vi "Pop-up Config.vi"(0 "Motor Pop-up Config":T1, 1 "Offset":T5, 2 "Motor Indicator":refnum<vi>, 3 "Motor Pop-up":refnum<vi>, 4 "VFD Pop-up":refnum<vi>, 5 "Motor_Title":refnum<vi>, 6 "Main Tab":refnum<vi>, 7 "VFD_Title":refnum<vi>, 9 "Motor Descriptions":string[](array[string]), 11 "Motor_Sel (Round)":refnum<vi>, 13 "Motor_Sel (Square)":refnum<vi>) -> ()   [LabVIEW 2020]
uses:
  <vilib>/Utility/miscctls.llb/LVPositionTypeDef.ctl
  Type Defs/Motor Pop-up Config Type Def.ctl
  Type Defs/Motors Type Def.ctl
  Type Defs/Motor Type Type Def.ctl
  Type Defs/Pop-up Corner Type Def.ctl
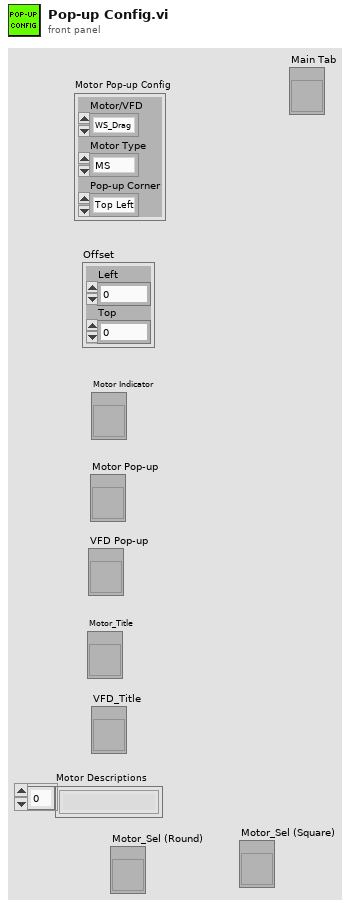
[diagram p1: front panel]
types:
  T1 = typedef "Motor Pop-up Config Type Def.ctl" = cluster{"Motor/VFD":T2, "Motor Type":T3, "Pop-up Corner":T4}
  T2 = typedef "Motors Type Def.ctl" = enum16{"WS_Drag", "WB_Drag", "WS_Fan", "WB_Fan", "Dryer_Drag", "Dryer_Fan", "DB_Fan", "DB_Drag", "DB_Top_Feed", "U-Trough", "Leg"}
  T3 = typedef "Motor Type Type Def.ctl" = enum16{"MS", "VFD"}
  T4 = typedef "Pop-up Corner Type Def.ctl" = enum16{"Top Left", "Top Right", "Bottom Left", "Bottom Right"}
  T5 = typedef "LVPositionTypeDef.ctl" = cluster{"Left":i32, "Top":i32}
  T6 = enum8{"Enabled", "Disabled", "Disabled and Grayed Out"}
  T7 = typedef "LVBoundsTypeDef.ctl" = cluster{"Width":u32, "Height":u32}
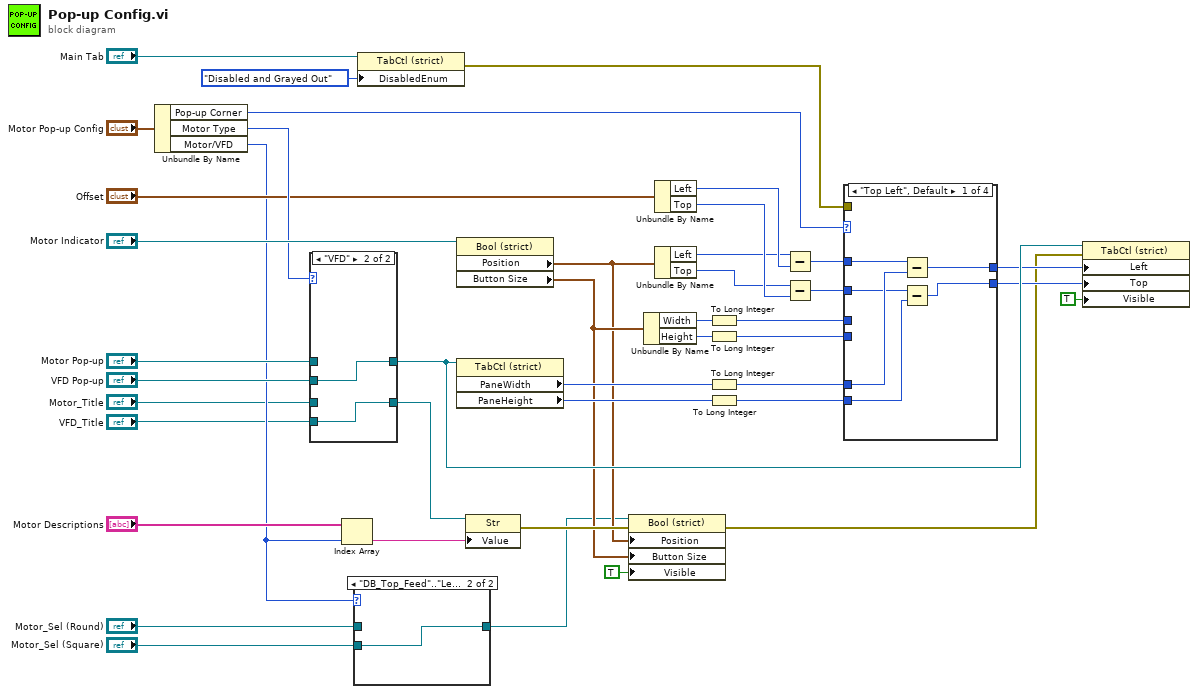
[diagram p0: block diagram]
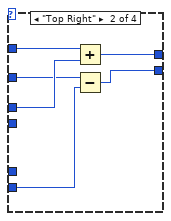
[diagram p4: hidden frame]
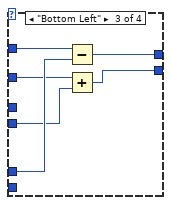
[diagram p5: hidden frame]
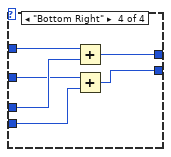
[diagram p6: hidden frame]
diagram:
  n1 = Unbundle By Name("Motor Pop-up Config") -> ("Pop-up Corner"=w16:T4, "Motor Type"=w33:T3, "Motor/VFD"=w6:T2)
  n2 = case shown="\"VFD\"" w33 {
    tunnel: [w44 w46] -> w38
    tunnel: "Motor Pop-up" -> [w44 _]
    tunnel: "VFD Pop-up" -> [_ w46]
    tunnel: [w43 w45] -> w42
    tunnel: "Motor_Title" -> [w43 _]
    tunnel: "VFD_Title" -> [_ w45]
    frame "MS", Default {
    }
    frame "VFD" {
    }
  }
  n3 = Index Array(array="Motor Descriptions", index=w6) -> (element=w41:string)
  n4 = case shown="\"DB_Top_Feed\"..\"Leg\"" w6 {
    tunnel: [w47 w48] -> w4
    tunnel: "Motor_Sel (Round)" -> [w47 _]
    tunnel: "Motor_Sel (Square)" -> [_ w48]
    frame Default {
    }
    frame "DB_Top_Feed".."Leg" {
    }
  }
  n5 = property on="Property Node" class="TabCtl (strict)"(reference="Main Tab", "DisabledEnum"=T6."Disabled and Grayed Out" ("Disabled")) -> (error out=w12:errorcluster)  [unwired: 1 in, 1 out]
  n6 = property on="Property Node" class="Bool (strict)"(reference="Motor Indicator") -> ("Position"=w8:T5, "Button Size"=w9:T7)  [unwired: 1 in, 2 out]
  n7 = property on="Property Node" class="TabCtl (strict)"(reference=w38) -> ("PaneWidth"=w35:u32, "PaneHeight"=w36:u32)  [unwired: 1 in, 2 out]
  n8 = property class="Str"(reference=w42, "Value"=w41) -> (error out=w11:errorcluster)  [unwired: 1 in, 1 out]
  n9 = property on="Property Node" class="Bool (strict)"(reference=w4, error in=w11, "Position"=w8, "Button Size"=w9, "Visible"=TRUE) -> (error out=w10:errorcluster)  [unwired: 1 out]
  n10 = Unbundle By Name(w9) -> ("Width"=w23:u32, "Height"=w24:u32)
  n11 = Unbundle By Name("Offset") -> ("Left"=w30:i32, "Top"=w31:i32)
  n12 = Unbundle By Name(w8) -> ("Left"=w28:i32, "Top"=w29:i32)
  n13 = To Long Integer(number=w23) -> (32bit integer=w22:i32)
  n14 = To Long Integer(number=w24) -> (32bit integer=w25:i32)
  n15 = To Long Integer(number=w35) -> (32bit integer=w21:i32)
  n16 = To Long Integer(number=w36) -> (32bit integer=w20:i32)
  n17 = Subtract(x=w28, y=w30) -> (x-y=w27:i32)
  n18 = Subtract(x=w29, y=w31) -> (x-y=w26:i32)
  n19 = case shown="\"Top Left\", Default" w16 {
    tunnel: [w54 w60 w66 w72] -> w18
    tunnel: [w53 w59 w65 w71] -> w19
    tunnel: w20 -> [w52 w58 _ _]
    tunnel: w21 -> [w51 _ w64 _]
    tunnel: w22 -> [_ w57 _ w69]
    tunnel: w25 -> [_ _ w63 w70]
    tunnel: w26 -> [w50 w55 w61 w67]
    tunnel: w27 -> [w49 w56 w62 w68]
    tunnel: w12 -> [_ _ _ _]
    frame "Top Left", Default {
      n20 = Subtract(x=w49, y=w51) -> (x-y=w54:i32)
      n21 = Subtract(x=w50, y=w52) -> (x-y=w53:i32)
    }
    frame "Top Right" {
      n22 = Add(x=w56, y=w57) -> (x+y=w60:i32)
      n23 = Subtract(x=w55, y=w58) -> (x-y=w59:i32)
    }
    frame "Bottom Left" {
      n24 = Subtract(x=w62, y=w64) -> (x-y=w66:i32)
      n25 = Add(x=w61, y=w63) -> (x+y=w65:i32)
    }
    frame "Bottom Right" {
      n26 = Add(x=w68, y=w69) -> (x+y=w72:i32)
      n27 = Add(x=w67, y=w70) -> (x+y=w71:i32)
    }
  }
  n28 = property on="Property Node" class="TabCtl (strict)"(reference=w38, error in=w10, "Left"=w18, "Top"=w19, "Visible"=TRUE) -> ()  [unwired: 2 out]
